vi "986x.Export.vi"(8 "error in (no error)":errorcluster, 11 "Device Item Ref in":T2 format="%.0x") -> (0 "error out":errorcluster, 2 "986x Support":T1, 3 "Item Ref out":T2 format="%.0x")   [LabVIEW 2019, in "Protection and Counter Addon System Explorer.lvlib"]
uses:
  Protection and Counter Addon System Explorer.lvlib
  <vilib>/NI VeriStand/Custom Device API/Custom Device Item Ref.ctl
  Shared/Types/986x.ctl
  Shared/SubVIs/GUID Lookup.vi
  <vilib>/NI VeriStand/Custom Device API/Get Item Property (Boolean).vi
  <vilib>/NI VeriStand/Custom Device API/Get Item Property (String).vi
  <vilib>/NI VeriStand/Custom Device API/Get Item Property (Dependent File).vi
  <vilib>/NI VeriStand/Custom Device API/Custom Device API.lvlib
  Shared/Protection and Counter Addon Shared.lvlib
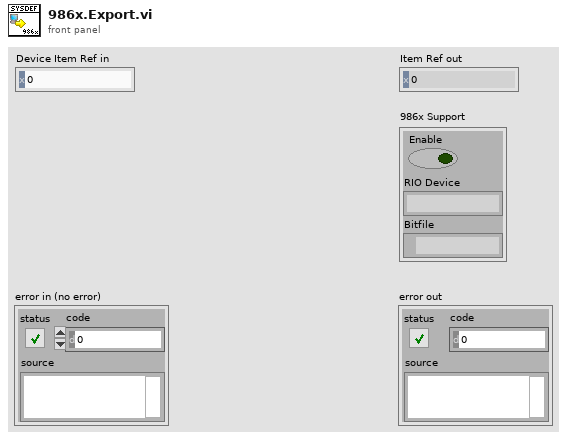
[diagram p1: front panel]
types:
  T1 = typedef "Protection and Counter Addon Shared.lvlib/986x.ctl" = cluster{"Enable":bool, "RIO Device":string, "Bitfile":path}
  T2 = typedef "Custom Device API.lvlib/Custom Device Item Ref.ctl" = u64
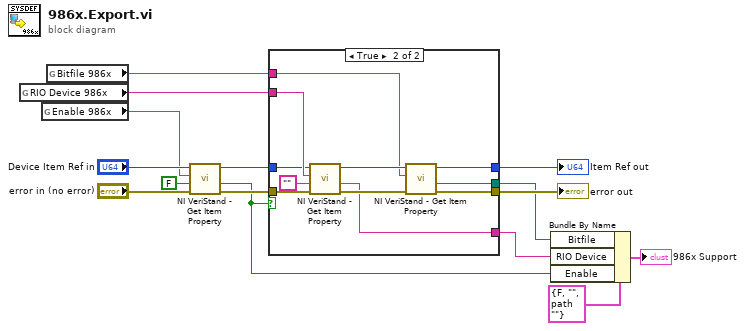
[diagram p0: block diagram]
diagram:
  n1 = global read "GUID Lookup.vi" "RIO Device 986x"() -> (w2:string)
  n2 = global read "GUID Lookup.vi" "Enable 986x"() -> (w3:string)
  n3 = global read "GUID Lookup.vi" "Bitfile 986x"() -> (w1:string)
  n4 = call-poly <vilib>:"NI VeriStand - Get Item Property.vi"("error in (no error)"="error in (no error)", "Default Value"=FALSE, "Property Name"=w3, "Item Ref in"="Device Item Ref in") -> ("error out"=w12:errorcluster, "Value"=w7:bool, "Item Ref out"=w13:T2)  [unwired: 4 in, 1 out]
  n5 = case shown="True" w7 {
    tunnel: w12 -> [w17 w28]
    tunnel: [w17 w25] -> w14
    tunnel: w2 -> [_ w27]
    tunnel: w1 -> [_ w23]
    tunnel: w13 -> [w16 w22]
    tunnel: [w16 w21] -> w15
    tunnel: [_ w20] -> w5
    tunnel: [_ w19] -> w6
    frame False {
    }
    frame True {
      n6 = call-poly <vilib>:"NI VeriStand - Get Item Property.vi"("error in (no error)"=w28, "Default Value"="", "Property Name"=w27, "Item Ref in"=w22) -> ("error out"=w26:errorcluster, "Value"=w20:string, "Item Ref out"=w24:T2)  [unwired: 4 in, 1 out]
      n7 = call-poly <vilib>:"NI VeriStand - Get Item Property.vi"("error in (no error)"=w26, "Property Name"=w23, "Item Ref in"=w24) -> ("error out"=w25:errorcluster, "Path"=w19:path, "Item Ref out"=w21:T2)  [unwired: 4 in, 2 out]
    }
  }
  "Item Ref out" <- w15
  "error out" <- w14
  n8 = Bundle By Name(cluster=T1 {"Enable"=FALSE, "RIO Device"="", "Bitfile"=path ""}, "Bitfile"=w6, "RIO Device"=w5, "Enable"=w7) -> (→"986x Support":T1)
